vi "TEMPLATE.vi"(7 "Is Sync":bool) -> (2 "Msg":refnum<class "Msg.lvclass">)   [LabVIEW 2021, in "_Template.lvlib" / "Templates.lvlib" / "TEMPLATE Msg.lvlib"]
uses:
  TEMPLATE Msg.lvlib
  jettl/jettl/Msg/Msg.lvclass
  TEMPLATE Msg/TEMPLATE Msg.lvclass
  C:/git/jettl/jettl/jettl/Msg/Msg.lvclass
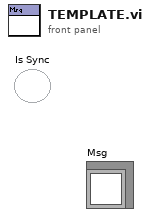
[diagram p1: front panel]
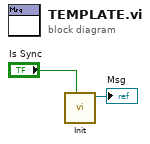
[diagram p0: block diagram]
diagram:
  n1 = call "Init.vi"("Is Sync"="Is Sync") -> ("TEMPLATE Msg out"=→"Msg":refnum<class "TEMPLATE Msg.lvclass">)  [unwired: 10 in]
